vi "Spartan HTTP Read Request.vi"(4 "error in (no error)":errorcluster, 7 "HTTP Session (empty)":T1 {"object data"."time" format="%0.2f"}) -> (0 "error out":errorcluster, 1 "Content Length":i32, 2 "HTTP Request":string, 3 "dup http session":T1 {"object data"."time" format="%0.2f"})   [LabVIEW 2011]
uses:
  Spartan HTTP Session.ctl
  ITK EXT/http/http_obj.llb/HTTP Session Data.ctl
  ITK EXT/utils/keyedarr.llb/Keyed Array.ctl
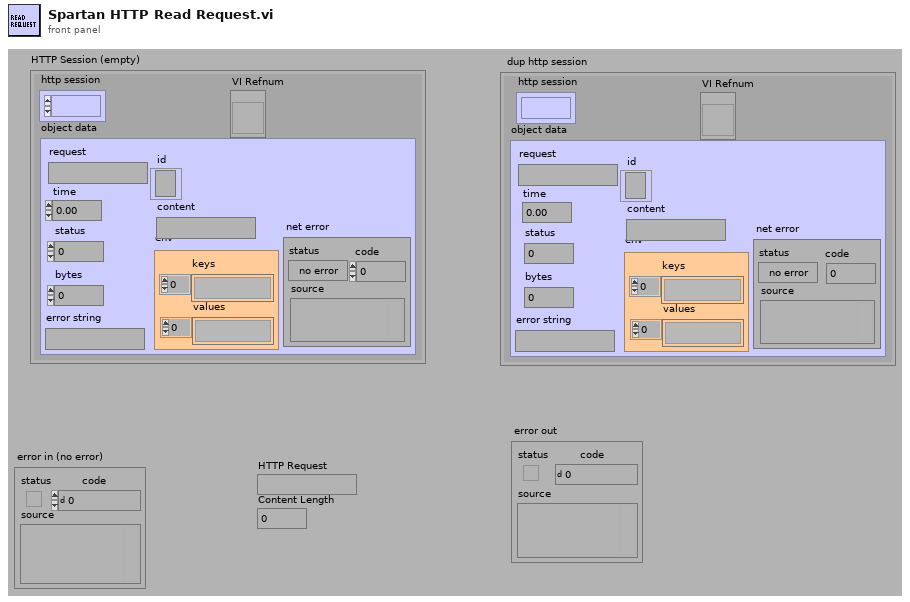
[diagram p1: front panel]
types:
  T1 = typedef "Spartan HTTP Session.ctl" = cluster{"http session":refnum<k1>, "object data":T2, "VI Refnum":refnum<vi>}
  T2 = typedef "HTTP Session Data.ctl" = cluster{"request":string, "time":dbl, "status":i32, "error string":string, "bytes":i32, "env":T3, "content":string, "id":refnum<k5>, "net error":errorcluster}
  T3 = typedef "Keyed Array.ctl" = cluster{"keys":string[], "values":string[]}
  T4 = enum16{"Standard", "Buffered", "CRLF", "Immediate"}
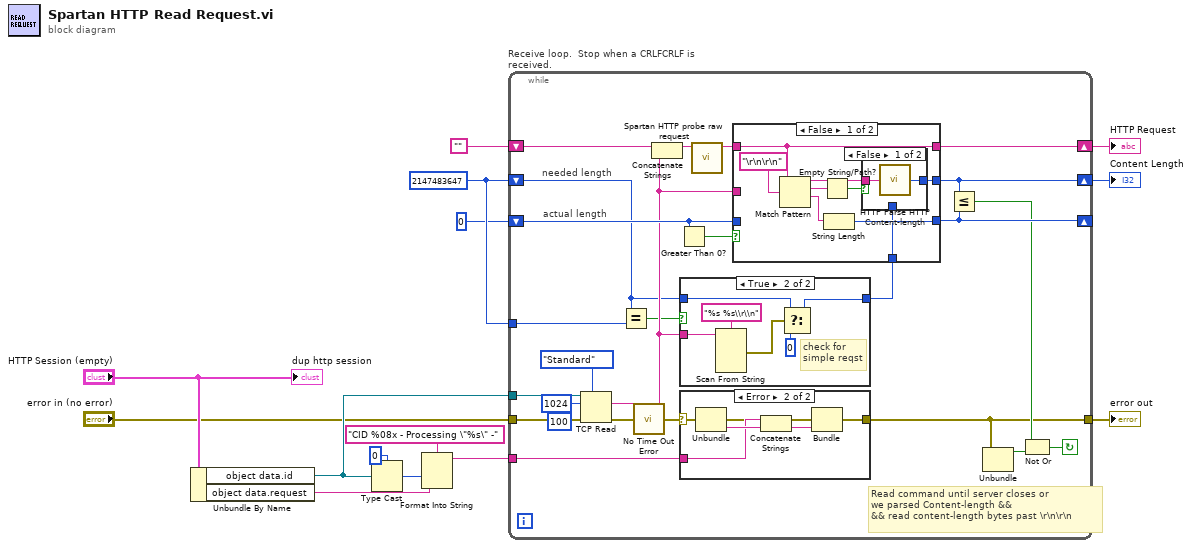
[diagram p0: block diagram]
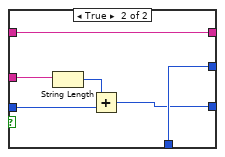
[diagram p5: hidden frame]
diagram:
  w13 = 2147483647
  n1 = Unbundle By Name("HTTP Session (empty)") -> ("object data.id"=w7:refnum<k5>, "object data.request"=w1:string)
  n2 = Type Cast(type=0, x=w7) -> (*(type *) &x=w6:i32)
  n3 = Format Into String(format string="CID %08x - Processing \"%s\" -", w6, w1) -> (resulting string=w4:string)  [unwired: 2 in, 1 out]
  n4 = while "Receive loop.  Stop when a CRLFCRLF is received." {
    tunnel: w13 -> [w28]
    shift-left: 0 -> [w34]
    shift-right: [w32] -> _
    shift-left: w13 -> [w26]
    shift-right: [w31] -> w10
    tunnel: "error in (no error)" -> [w36]
    shift-left: "" -> [w33]
    shift-right: [w39] -> w11
    tunnel: [w21] -> w9
    tunnel: w7 -> [w17]
    tunnel: w4 -> [w24]
    stop <- w38 continue-if-true
    # "Read command until server closes or\nwe parsed Content-length &&\n&& read content-length bytes past \\r\\n\\r\\n"
    # "needed length"
    # "actual length"
    n5 = TCP Read(connection ID=w17, bytes to read=1024, error in (no error)=w36, 7:T4."Standard" ("mode (standard)"), 9:100 ("timeout ms (25000)")) -> (data out=w29:string, error out=w20:errorcluster)  [unwired: 1 out]
    n6 = Equal?(x=w26, y=w28) -> (x = y?=w27:bool)
    n7 = call "No Time Out Error.vi"("error in (no error)"=w20) -> ("error out"=w19:errorcluster)  [unwired: 14 out]
    n8 = Concatenate Strings(w33, w29) -> (w23:string)
    n9 = Greater Than 0?(x=w34) -> (x > 0?=w35:bool)
    n10 = case shown="True" w27 {
      tunnel: w29 -> [_ w51]
      tunnel: w26 -> [w46 w50]
      tunnel: [w46 w48] -> w25
      frame False {
        # "we have a simple request\nor we know the size"
      }
      frame True {
        # "check for\nsimple reqst"
        n11 = Scan From String(format string="%s %s\\r\\n", input string=w51) -> (error out=w47:errorcluster)  [unwired: 2 in, 6 out]
        n12 = Select(t=w50, s=w47, f=0) -> (s? t:f=w48:i32)
      }
    }
    n13 = case shown="Error" w19 {
      selector: w19 -> [w40 w43]
      tunnel: [w40 w42] -> w21
      tunnel: w24 -> [_ w44]
      frame No Error {
      }
      frame Error {
        n14 = Unbundle(w43) -> ("source"=w45:string)  [unwired: 2 out]
        n15 = Concatenate Strings(w44, w45) -> (w41:string)
        n16 = Bundle(cluster=w43, "source"=w41) -> (w42:errorcluster)  [unwired: 2 out]
      }
    }
    n17 = call "Spartan HTTP probe raw request.vi"("Request"=w23) -> ("dup Request"=w22:string)  [unwired: 10 out]
    n18 = case shown="False" w35 {
      tunnel: w29 -> [_ w68]
      tunnel: w22 -> [w60 w70]
      tunnel: [w60 w70] -> w39
      tunnel: [w58 w69] -> w31
      tunnel: w25 -> [w55 w69]
      tunnel: [w56 w67] -> w32
      tunnel: w34 -> [_ w65]
      frame False {
        n19 = Match Pattern(string=w60, regular expression="\r\n\r\n") -> (before substring=w59:string, match substring=w53:string, after substring=w57:string)  [unwired: 2 out]
        n20 = Empty String/Path?(string/path=w53) -> (empty?=w54:bool)
        n21 = String Length(string=w57) -> (length=w56:i32)
        n22 = case shown="False" w54 {
          tunnel: [w63 w64] -> w58
          tunnel: w59 -> [w62 _]
          tunnel: w55 -> [_ w64]
          frame False {
            n23 = call "HTTP Parse HTTP Content-length.vi"("HTTP Command"=w62) -> ("Content-length"=w63:i32)
          }
          frame True {
          }
        }
      }
      frame True {
        n24 = String Length(string=w68) -> (length=w66:i32)
        n25 = Add(x=w66, y=w65) -> (x+y=w67:i32)
      }
    }
    n26 = Less Or Equal?(x=w31, y=w32) -> (x <= y?=w30:bool)
    n27 = Unbundle(w21) -> ("status"=w37:bool)  [unwired: 2 out]
    n28 = Not Or(1:w37, 2:w30) -> (0:w38:bool)
  }
  "error out" <- w9
  "HTTP Request" <- w11
  "Content Length" <- w10
  "dup http session" <- "HTTP Session (empty)"
